vi "loadCalibrationData.vi"(10 "DAQmx \nPhysical Channel":tag="Dev2/ai0:31") -> (0 "channel names out":string[](array[string]), 1 "zeroSignals":dbl[](array[numeric]), 2 "voltsPerGram":dbl[](array[numeric]), 3 "index":i32[](array[numeric]))   [LabVIEW 2017]
panel:
  # "Channels to weigh"
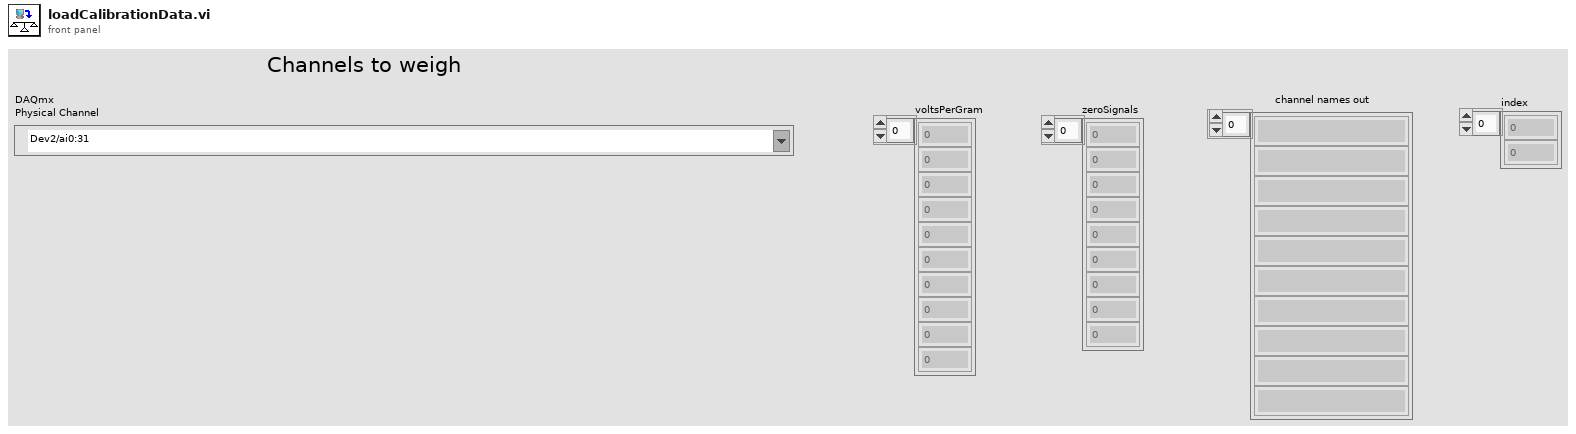
[diagram p1: front panel]
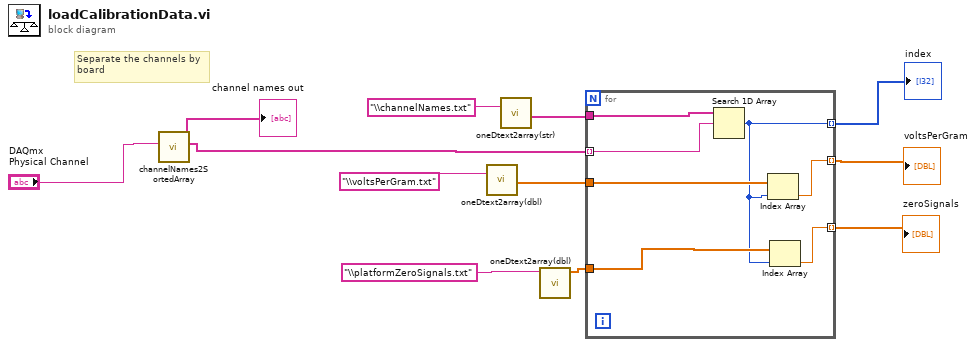
[diagram p0: block diagram]
diagram:
  # "Separate the channels by\nboard"
  n1 = call "channelNames2SortedArray.vi"("DAQmx \nPhysical Channel"="DAQmx \nPhysical Channel") -> ("names out"=w2:string[])  [unwired: 10 in]
  "channel names out" <- w2
  n2 = call "oneDtext2array(dbl).vi"("String"="\\voltsPerGram.txt") -> ("array"=w7:dbl[])  [unwired: 10 in]
  n3 = call "oneDtext2array(str).vi"("String"="\\channelNames.txt") -> ("text"=w9:string[])  [unwired: 10 in]
  n4 = call "oneDtext2array(dbl).vi"("String"="\\platformZeroSignals.txt") -> ("array"=w4:dbl[])  [unwired: 10 in]
  n5 = for {
    tunnel: w2 -> [w18] mode=indexing
    tunnel: w9 -> [w17]
    tunnel: w4 -> [w16]
    tunnel: [w15] -> w11 mode=indexing
    tunnel: [w14] -> w8 mode=indexing
    tunnel: w7 -> [w13]
    tunnel: [w12] -> w1 mode=indexing
    n6 = Search 1D Array(1D array=w17, element=w18) -> (index of element=w12:i32)  [unwired: 1 in]
    n7 = Index Array(array=w13, index=w12) -> (element=w14:dbl)
    n8 = Index Array(array=w16, index=w12) -> (element=w15:dbl)
  }
  "voltsPerGram" <- w8
  "zeroSignals" <- w11
  "index" <- w1
